vi "FGV - Initialise.vi"(0 "Enum":T1=enum."Get Data", 1 "DAQ - Task IN":refnum<k21>, 2 "simulator":refnum<class "dotnet_system_exec.lvclass">, 3 "connection ID":refnum<k16>, 4 "Handle In":u64, 5 "Error In":errorcluster) -> (15 "task out":refnum<k21>, 16 "simulator":refnum<class "dotnet_system_exec.lvclass">, 17 "connection ID":refnum<k16>, 18 "Handle Out":u64, 19 "Error Out":errorcluster)   [LabVIEW 2024]
doc: "Uses an enum to control the action.\nInitilise the I2C and DAQ devices. \nIt also reads the handle of these devices \nCan clean up the I2C and DAQ at end of the test"
uses:
  <vilib>/JKI/JKI DotNet System Exec/dotnet_system_exec/dotnet_system_exec.lvclass
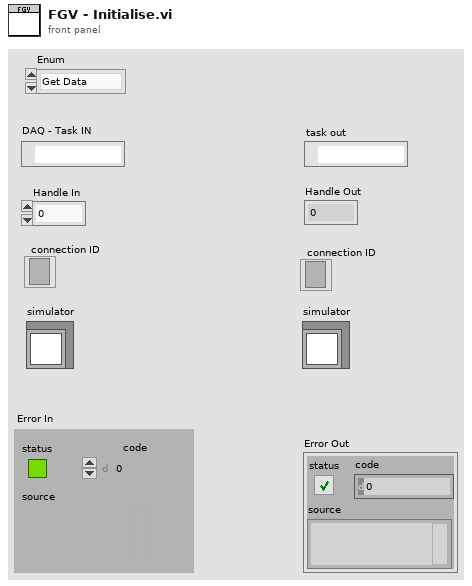
[diagram p1: front panel]
types:
  T1 = typedef "FGV - Enum" = enum16{"Cleanup", "Get Data", "Simulator", "Open UDP", "Initialise DAQ", "Initialise I2C"}
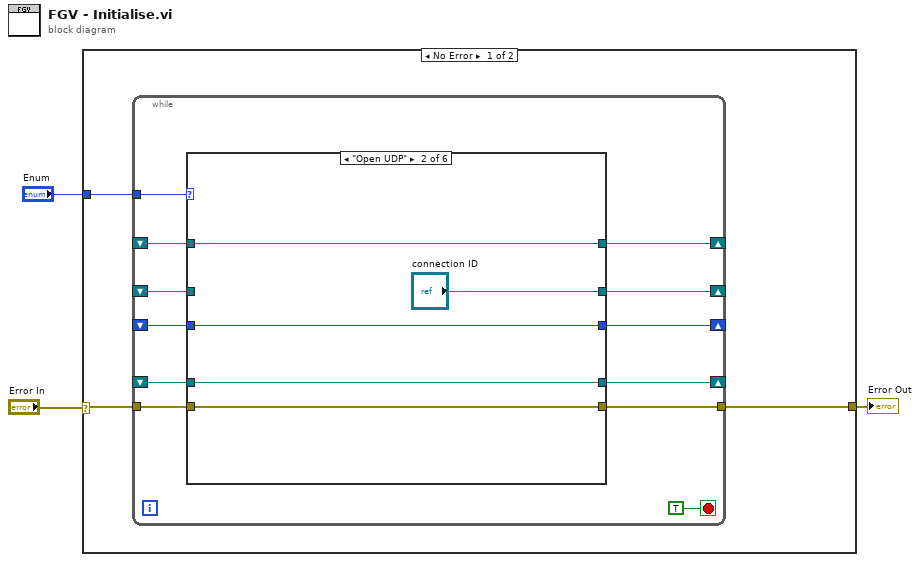
[diagram p0: block diagram]
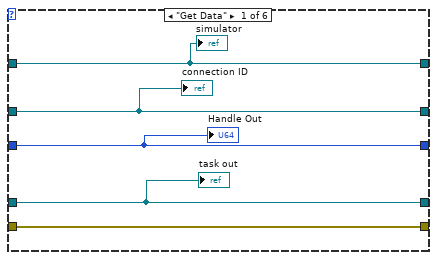
[diagram p2: hidden frame]
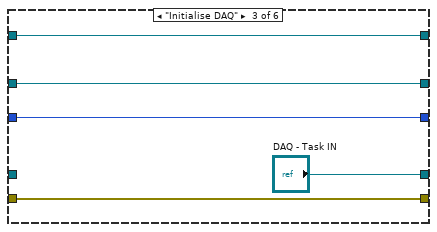
[diagram p3: hidden frame]
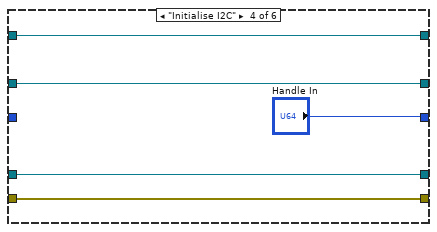
[diagram p4: hidden frame]
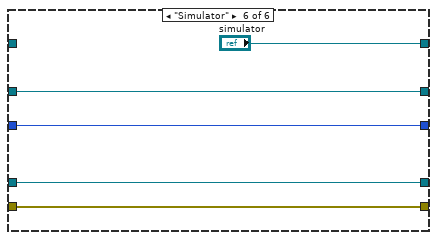
[diagram p6: hidden frame]
diagram:
  n1 = case shown="No Error" "Error In" {
    selector: "Error In" -> [w4 w49]
    tunnel: "Enum" -> [w6 _]
    tunnel: [w5 w49] -> w1
    frame No Error {
      n2 = while {
        tunnel: w6 -> [w17]
        tunnel: [w16] -> w5
        tunnel: w4 -> [w15]
        shift-right: [w14] -> _
        shift-left: _ -> [w11]
        shift-right: [w13] -> _
        shift-left: _ -> [w12]
        shift-right: [w10] -> _
        shift-left: _ -> [w9]
        shift-right: [w8] -> _
        shift-left: _ -> [w7]
        stop <- TRUE stop-if-true
        n3 = case shown="\"Open UDP\"" w17 {
          tunnel: [w23 w28 w31 w36 w41 w44] -> w16
          tunnel: w15 -> [w23 w28 w31 w36 w41 w44]
          tunnel: [w20 w27 "DAQ - Task IN" w37 w42 w45] -> w14
          tunnel: [w21 w26 w32 "Handle In" w43 w46] -> w13
          tunnel: w12 -> [w21 w26 w32 _ w43 w46]
          tunnel: w11 -> [w20 w27 _ w37 w42 w45]
          tunnel: [w22 "connection ID" w30 w35 w40 w47] -> w10
          tunnel: w9 -> [w22 _ w30 w35 w40 w47]
          tunnel: [w19 w24 w29 w34 w39 "simulator"] -> w8
          tunnel: w7 -> [w19 w24 w29 w34 w39 _]
          frame "Get Data" {
            "connection ID" <- w22
            "Handle Out" <- w21
            "task out" <- w20
            "simulator" <- w19
          }
          frame "Open UDP" {
          }
          frame "Initialise DAQ" {
          }
          frame "Initialise I2C" {
          }
          frame "Cleanup" {
          }
          frame "Simulator" {
          }
        }
      }
    }
    frame Error {
    }
  }
  "Error Out" <- w1
